vi "Keysight handler.vi"(8 "error in (no error)":errorcluster, 11 "Message Queues out":T1) -> (0 "error out":errorcluster, 3 "Message Queue":refnum<queue>)   [LabVIEW 2014]
uses:
  support/Message Queue/Message Queue.lvlib
  support/Message Queue/Enqueue Message (Single).vi
  <vilib>/ErrorRing/Error Ring.xnode
  support/Message Queue/Lossy Enqueue Message (Single).vi
  <vilib>/Utility/error.llb/Error Cluster From Error Code.vi
  Laser/Keyence data cluster.ctl
  Multimeter settings.ctl
  <instrlib>/Agilent 3446X Series/Public/Data/Read (Single Point).vi
  <vilib>/ethernetip/ethernetip.llb/ethernetip.ctl
  <vilib>/ethernetip/ethernetip.lvlib
  support/Message Queue/Message Cluster.ctl
  support/Message Queue/All Message Queues.ctl
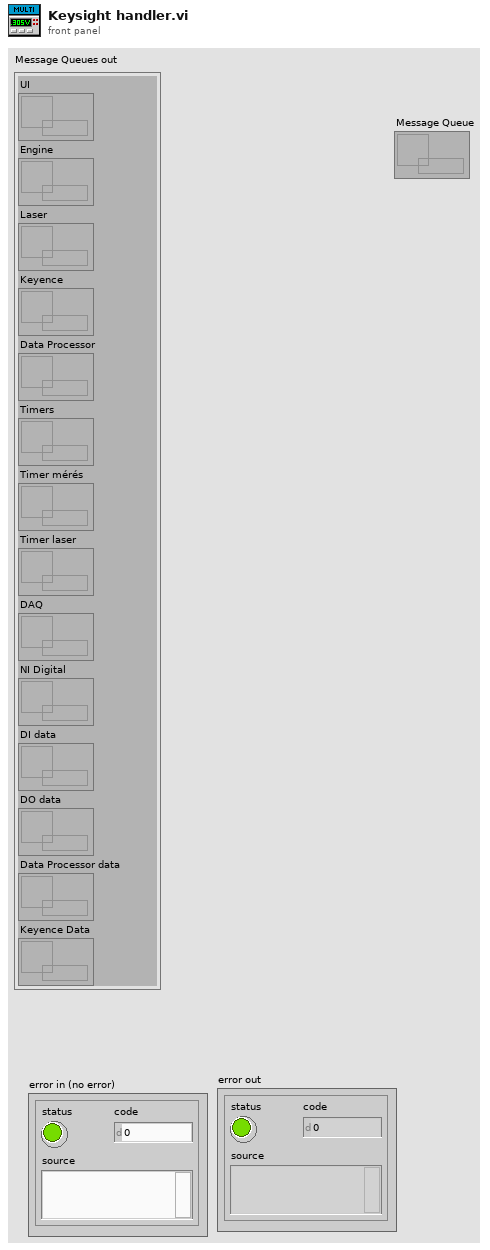
[diagram p1: front panel]
types:
  T1 = typedef "Message Queue.lvlib/All Message Queues.ctl" = cluster{"UI":refnum<queue>, "Engine":refnum<queue>, "Laser":refnum<queue>, "Keyence":refnum<queue>, "Data Processor":refnum<queue>, "Timers":refnum<queue>, "Timer mérés":refnum<queue>, "Timer laser":refnum<queue>, "DAQ":refnum<queue>, "NI Digital":refnum<queue>, "DI data":refnum<queue>, "DO data":refnum<queue>, "Data Processor data":refnum<queue>, "Keyence Data":refnum<queue>}
  T2 = typedef "Keyence data cluster.ctl" = cluster{"Communication Opened":bool, "Result":dbl[], "Read":bool, "Ethernet/IP Session":T3, "Ethernet/IP parameters":cluster{"IP":string, "Class":dbl, "Attribute":dbl, "Get Instance":dbl, "Set Instance":dbl}}
  T3 = typedef "ethernetip.lvlib/ethernetip.ctl" = refnum<k21>
  T4 = typedef "Multimeter settings.ctl" = cluster{"Measurement Function (10: Voltage DC)":i32, "Absolute Resolution (1E-6)":dbl, "Auto Range (T: Enable)":bool, "Manual Range (1)":dbl, "Command":string}
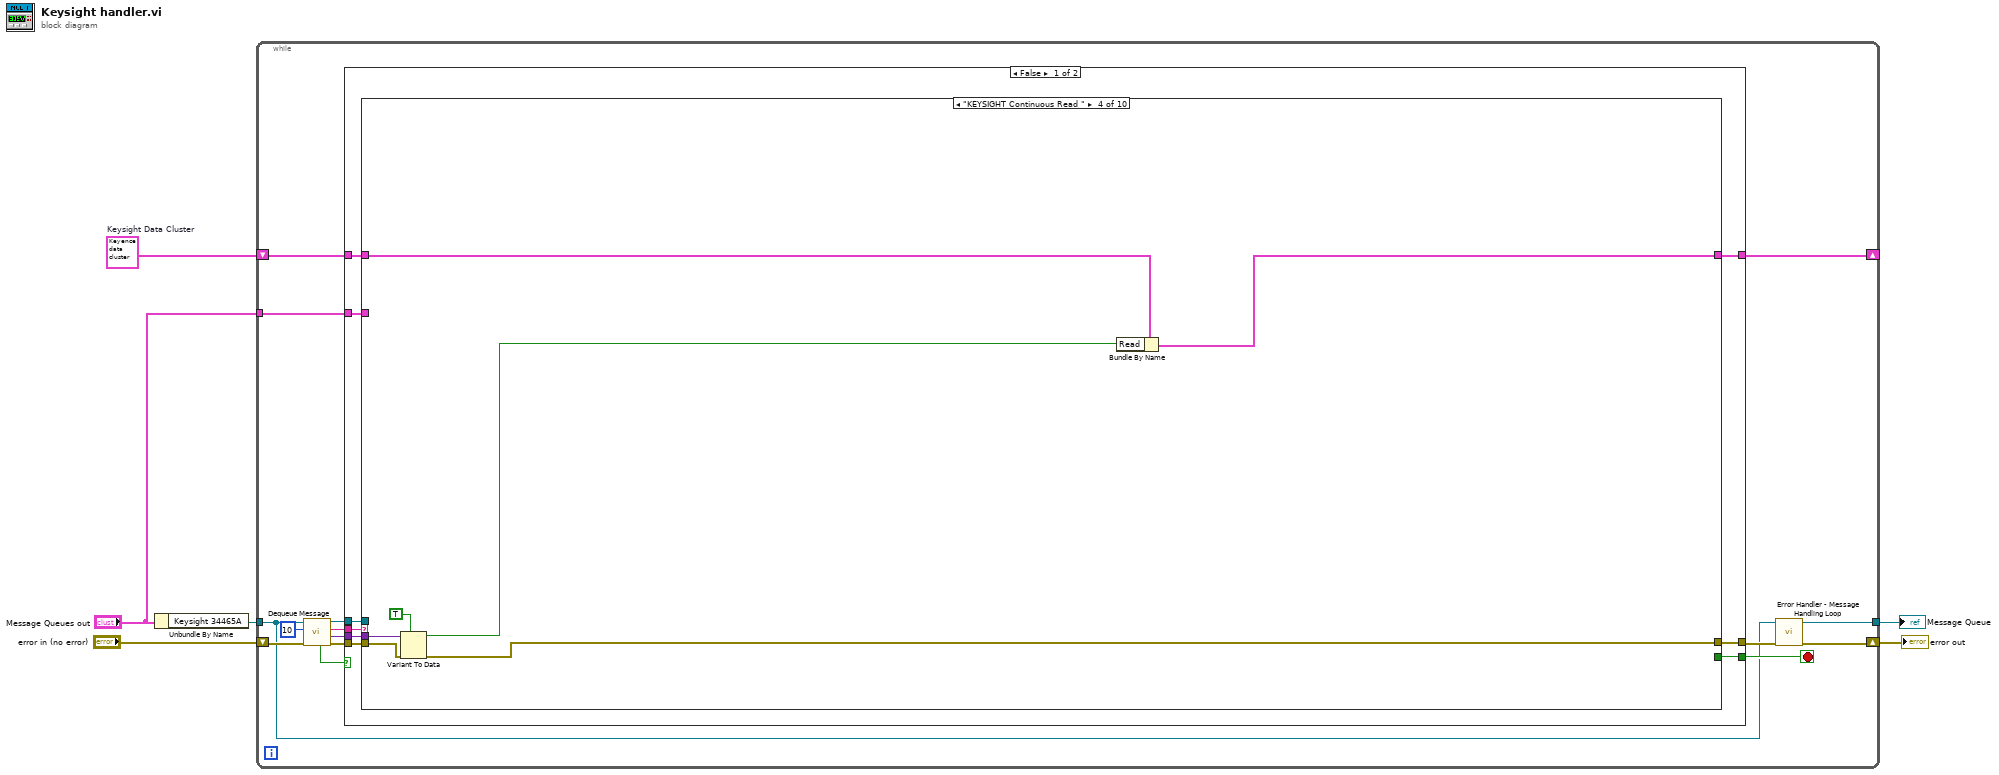
[diagram p0: block diagram]
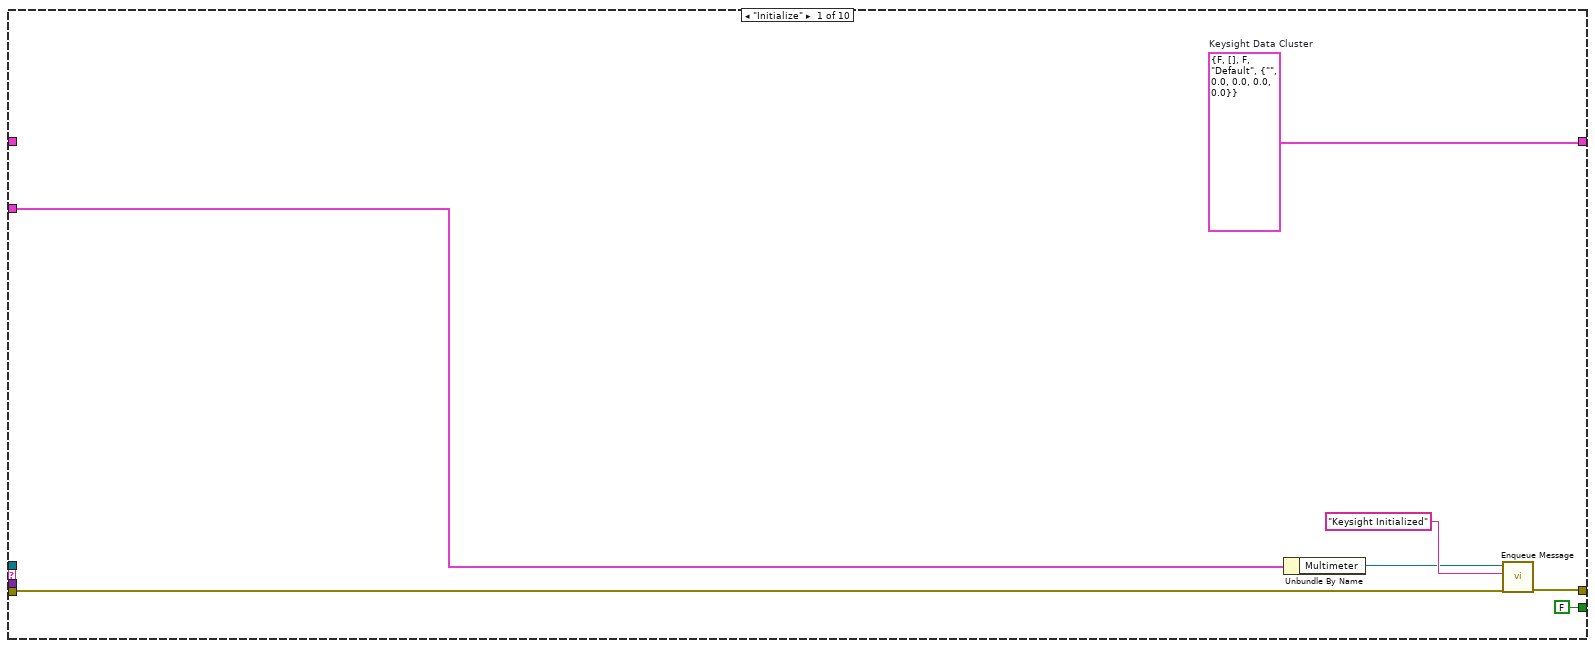
[diagram p2: hidden frame]
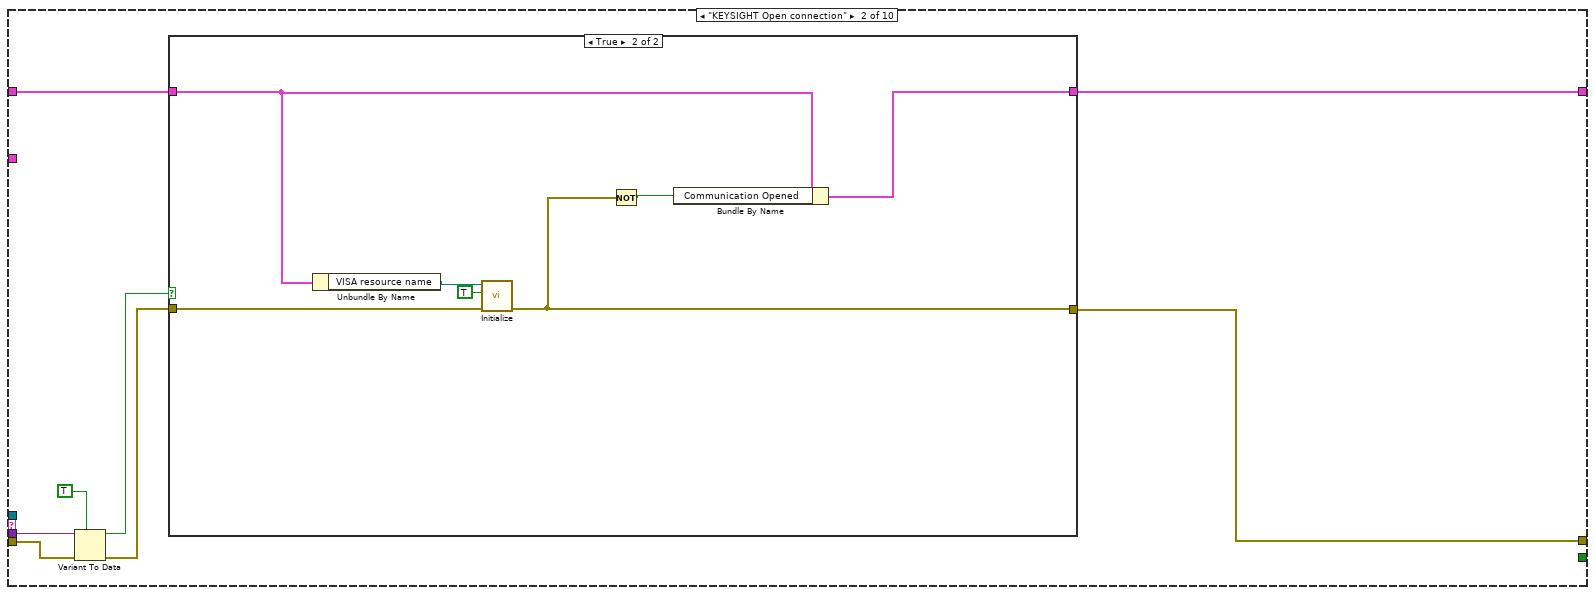
[diagram p3: hidden frame]
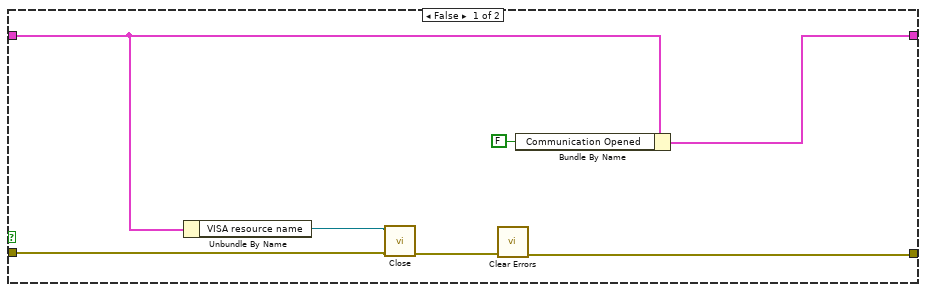
[diagram p4: hidden frame]
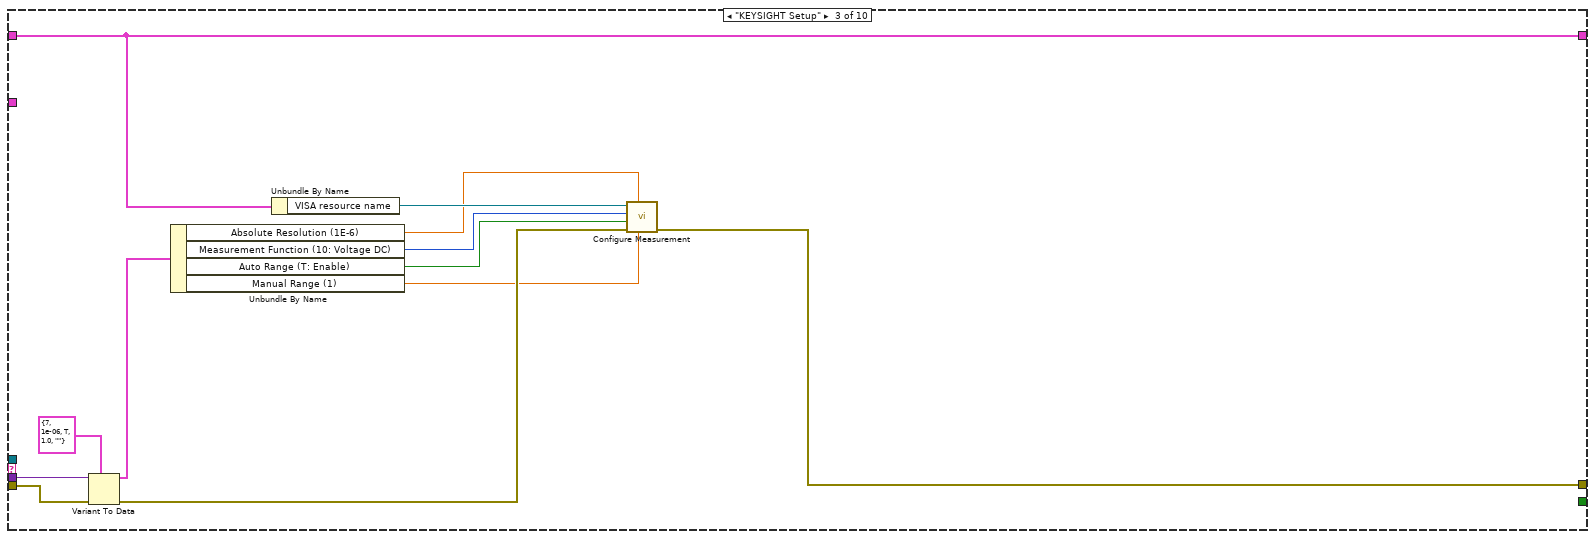
[diagram p5: hidden frame]
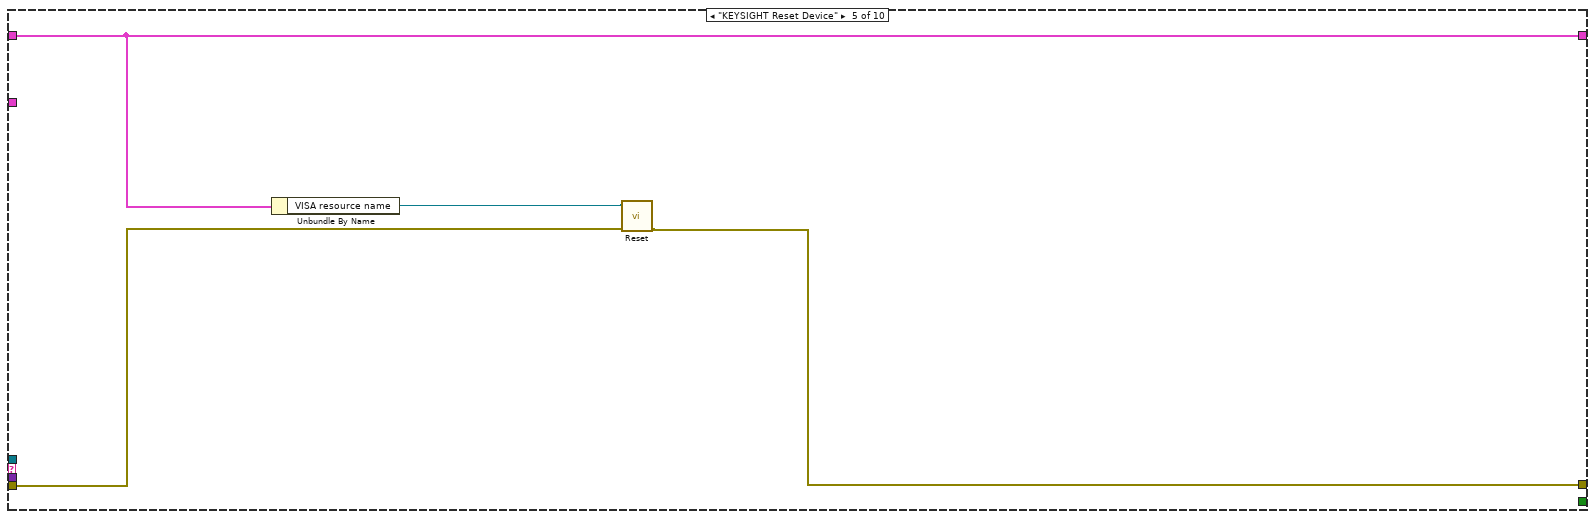
[diagram p6: hidden frame]
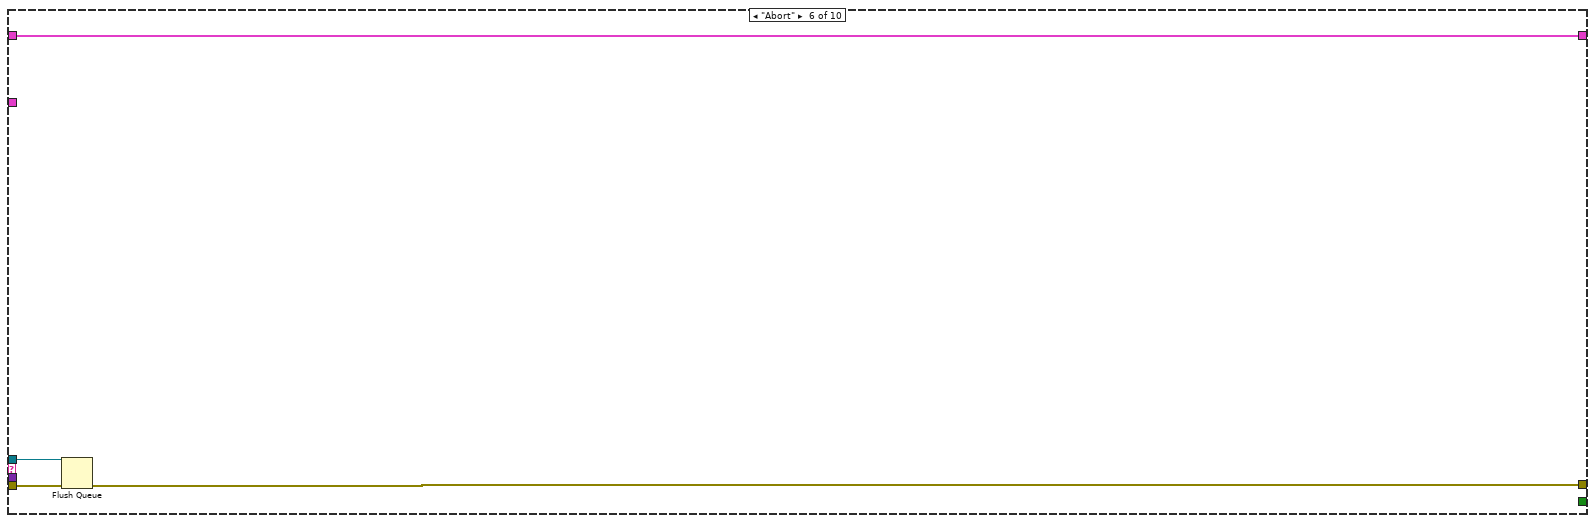
[diagram p7: hidden frame]
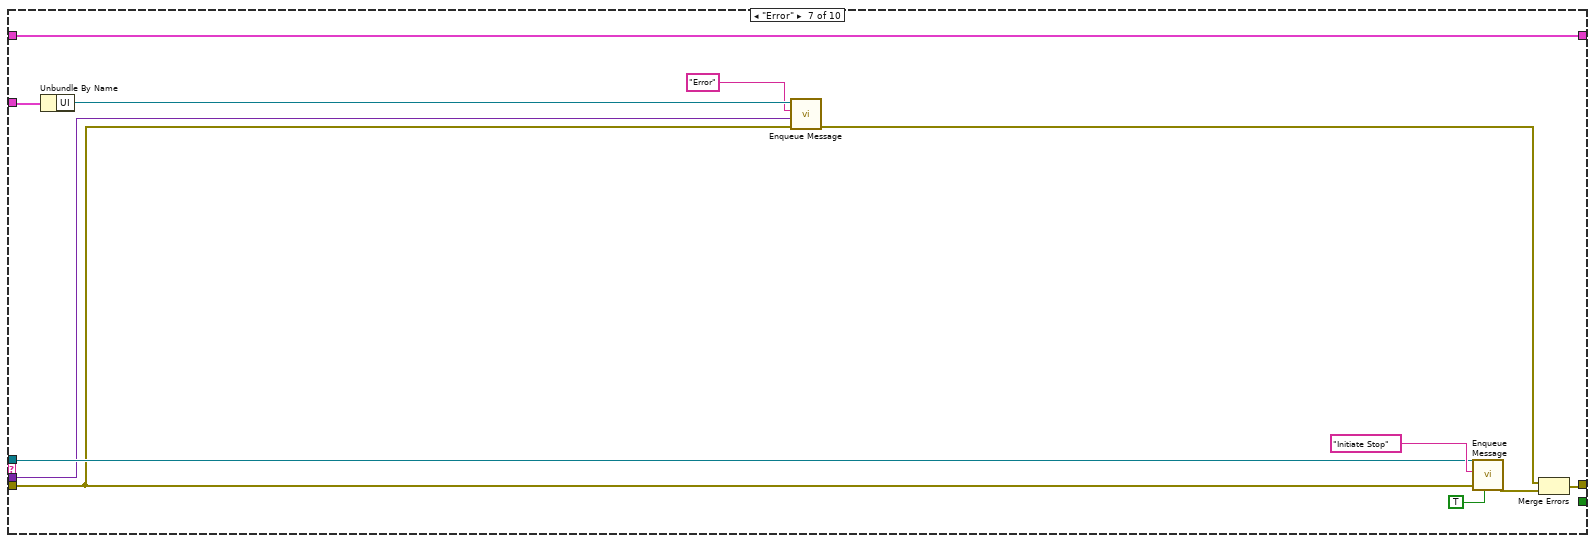
[diagram p8: hidden frame]
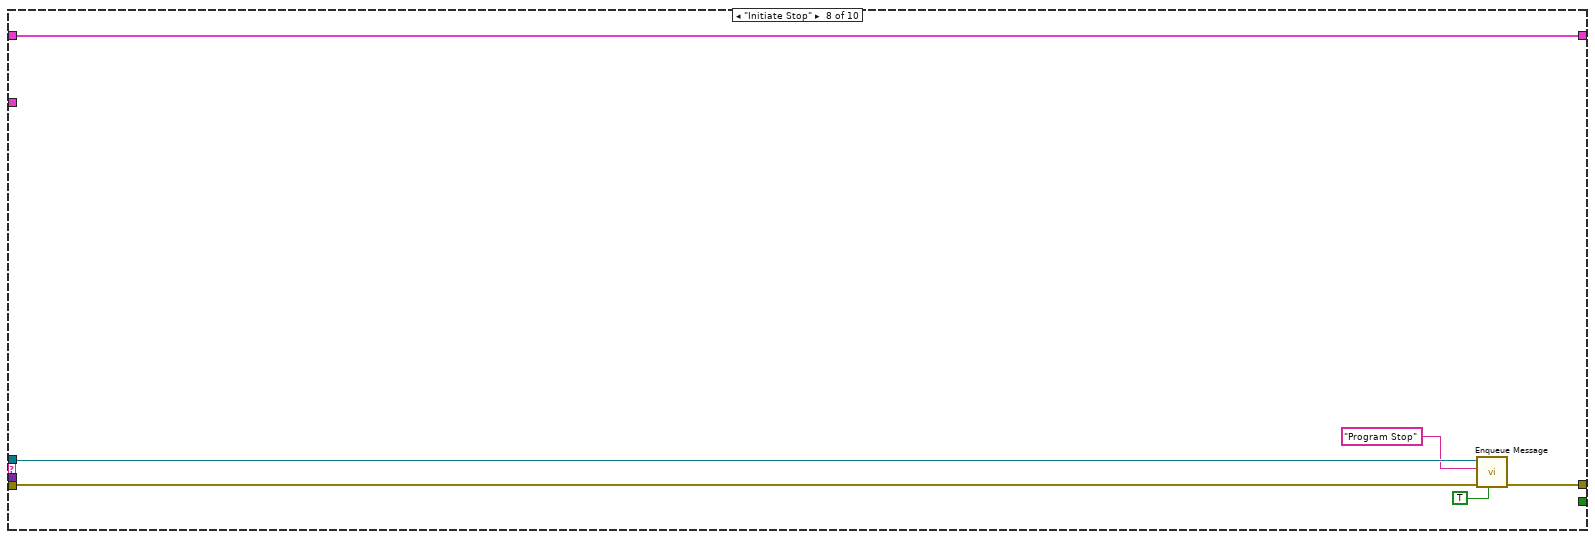
[diagram p9: hidden frame]
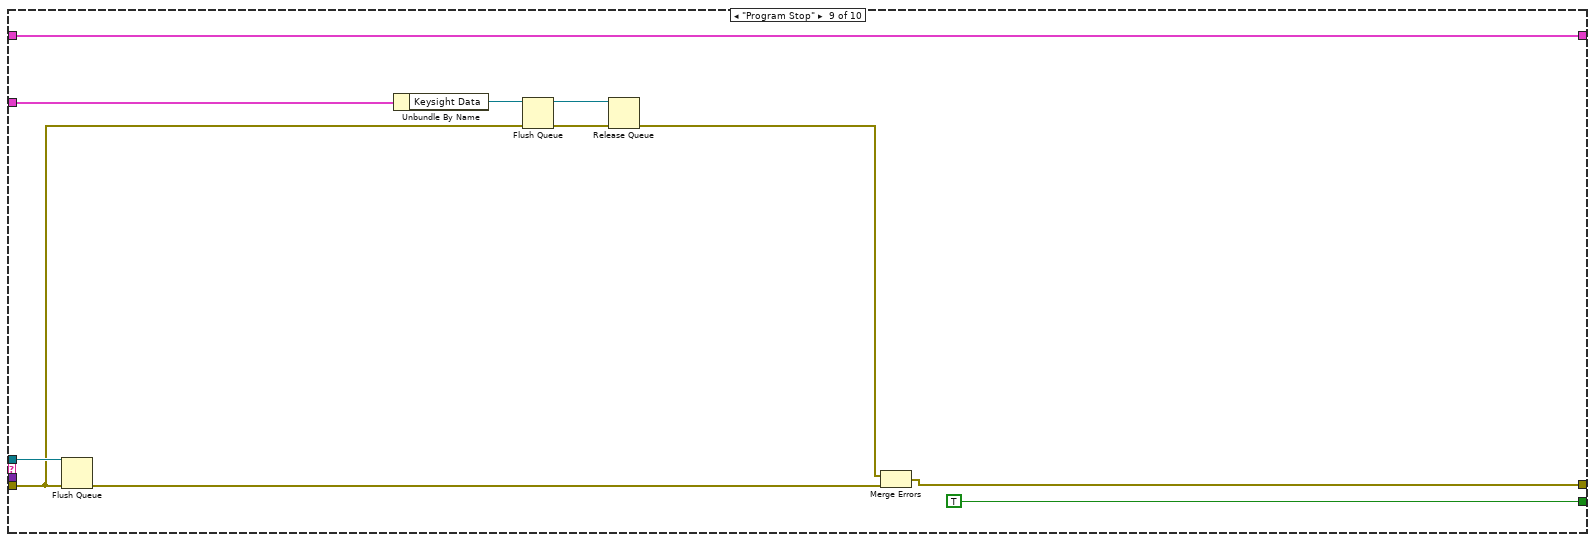
[diagram p10: hidden frame]
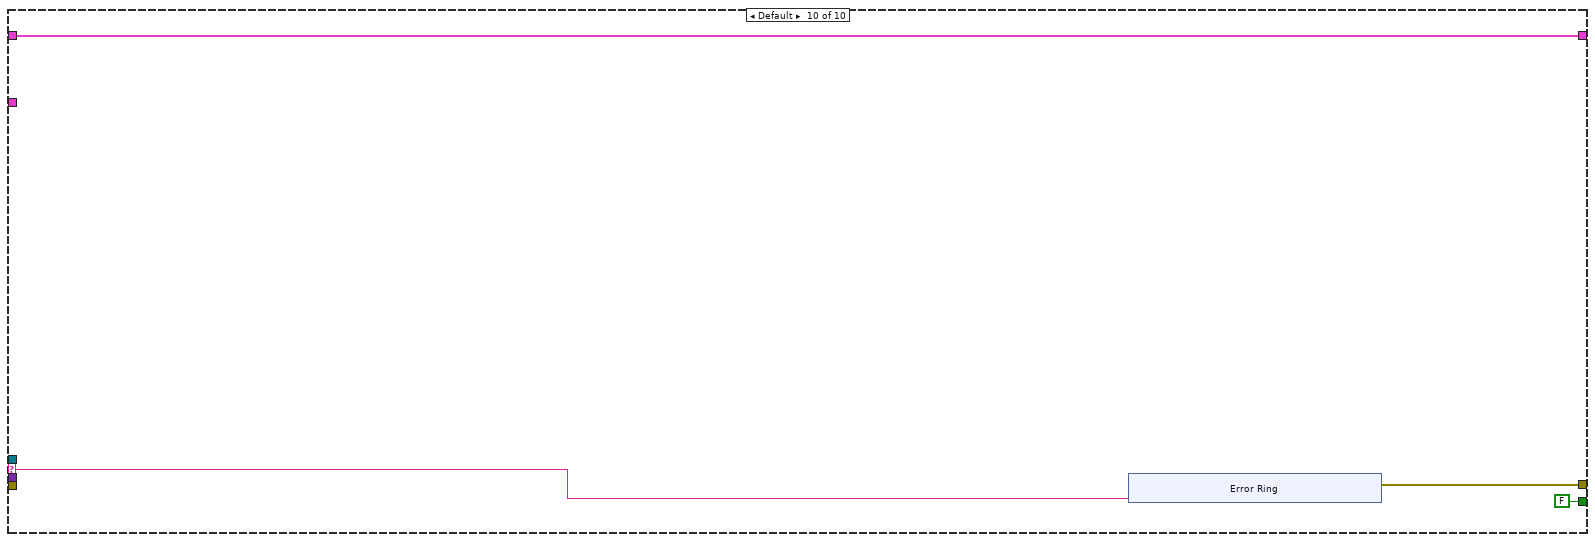
[diagram p11: hidden frame]
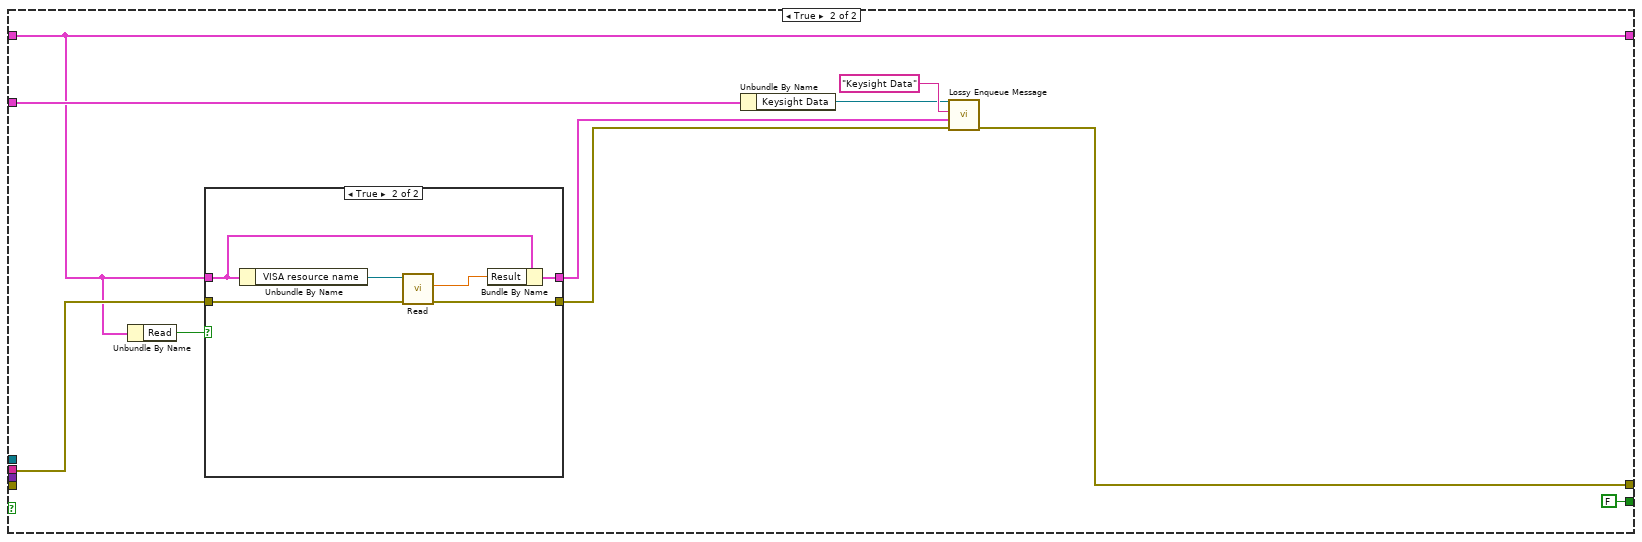
[diagram p12: hidden frame]
diagram:
  w1 = T2 {"Communication Opened"=FALSE, "Result"=[], "Read"=FALSE, "Ethernet/IP Session"="Default", "Ethernet/IP parameters"={"IP"="", "Class"=0.0, "Attribute"=0.0, "Get Instance"=0.0, "Set Instance"=0.0}}  # Keysight Data Cluster
  n1 = Unbundle By Name("Message Queues out") -> ("Keysight 34465A"=w3:refnum<queue>)
  n2 = while {
    tunnel: w3 -> [w7]
    shift-right: [w8] -> _
    shift-left: w1 -> [w14]
    shift-right: [w12] -> w6
    shift-left: "error in (no error)" -> [w21]
    tunnel: "Message Queues out" -> [w10]
    tunnel: [w9] -> w2
    stop <- w17 stop-if-true
    n3 = call "Dequeue Message.vi"("error in (no error)"=w21, "timeout in ms (-1)"=10, "Message Queue"=w7) -> ("error out"=w19:errorcluster, "Message Data"=w13:variant, "Message"=w20:string, "dup Message Queue"=w18:refnum<queue>, "timed out?"=w15:bool)  [unwired: 4 in]
    n4 = case shown="False" w15 {
      tunnel: w20 -> [w30 _]
      tunnel: w19 -> [w29 w131]
      tunnel: w18 -> [w28 _]
      tunnel: [w27 FALSE] -> w17
      tunnel: [w26 w132] -> w11
      tunnel: w14 -> [w24 w128]
      tunnel: [w25 w128] -> w8
      tunnel: w13 -> [w23 _]
      tunnel: w10 -> [w22 w133]
      frame False {
        n5 = case shown="\"KEYSIGHT Continuous Read \"" w30 {
          selector: w30 -> [_ _ _ _ _ _ _ _ _ w116]
          tunnel: w29 -> [w32 w41 w70 w75 w82 w86 w88 w102 w105 _]
          tunnel: w28 -> [_ _ _ _ _ w85 w91 w101 w115 _]
          tunnel: [w36 w38 w61 w72 w80 w83 w92 w103 w106 w117] -> w26
          tunnel: [FALSE _ _ _ _ _ _ _ TRUE FALSE] -> w27
          tunnel: [w31 w39 w60 w77 w79 w84 w87 w104 w113 w119] -> w25
          tunnel: w24 -> [_ w40 w60 w78 w79 w84 w87 w104 w113 w119]
          tunnel: w23 -> [_ w42 w71 w76 _ _ w89 _ _ _]
          tunnel: w22 -> [w33 _ _ _ _ _ w90 _ w108 _]
          frame "Initialize" {
            w31 = T2 {"Communication Opened"=FALSE, "Result"=[], "Read"=FALSE, "Ethernet/IP Session"="Default", "Ethernet/IP parameters"={"IP"="", "Class"=0.0, "Attribute"=0.0, "Get Instance"=0.0, "Set Instance"=0.0}}  # Keysight Data Cluster
            n6 = Unbundle By Name(w33) -> ("Multimeter"=w34:refnum<queue>)
            n7 = call-poly "Enqueue Message.vi"("error in (no error)"=w32, "Message"="Keysight Initialized", "Message Queue"=w34) -> ("error out"=w36:errorcluster)  [unwired: 7 in, 1 out]
          }
          frame "KEYSIGHT Open connection" {
            n8 = Variant To Data(error in=w41, type=TRUE ("Control word.Enable Voltage"), Variant=w42) -> (data=w43:bool, error out=w44:errorcluster)
            n9 = case shown="True" w43 {
              tunnel: w44 -> [w48 w59]
              tunnel: w40 -> [w52 w57]
              tunnel: [w50 w54] -> w38
              tunnel: [w49 w56] -> w39
              frame False {
                n10 = Unbundle By Name(w52) -> ("VISA resource name"=w46:refnum<visa-resource-name>)
                n11 = call <instrlib>:"Close.vi"("error in (no error)"=w48, "VISA resource name"=w46) -> ("error out"=w47:errorcluster)  [unwired: 9 in]
                n12 = call <vilib>:"Clear Errors.vi"("error in (no error)"=w47) -> ("error out"=w50:errorcluster)  [unwired: 5 in, 1 out]
                n13 = Bundle By Name(cluster=w52, "Communication Opened"=FALSE) -> (w49:T2)
              }
              frame True {
                n14 = Unbundle By Name(w57) -> ("VISA resource name"=w58:refnum<visa-resource-name>)
                n15 = call <instrlib>:"Initialize.vi"("error in (no error)"=w59, "ID Query (True)"=TRUE, "VISA resource name"=w58) -> ("error out"=w54:errorcluster)  [unwired: 7 in, 1 out]
                n16 = Not(x=w54) -> (.not. x?=w55:bool)
                n17 = Bundle By Name(cluster=w57, "Communication Opened"=w55) -> (w56:T2)
              }
            }
          }
          frame "KEYSIGHT Setup" {
            n18 = Variant To Data(error in=w70, type=T4 {"Measurement Function (10: Voltage DC)"=7, "Absolute Resolution (1E-6)"=1e-06, "Auto Range (T: Enable)"=TRUE, "Manual Range (1)"=1.0, "Command"=""} ("Multimeter settings"), Variant=w71) -> (data=w68:T4, error out=w66:errorcluster)
            n19 = Unbundle By Name(w68) -> ("Absolute Resolution (1E-6)"=w65:dbl, "Measurement Function (10: Voltage DC)"=w64:i32, "Auto Range (T: Enable)"=w63:bool, "Manual Range (1)"=w62:dbl)
            n20 = Unbundle By Name(w60) -> ("VISA resource name"=w67:refnum<visa-resource-name>)
            n21 = call <instrlib>:"Configure Measurement.vi"("Manual Range (1)"=w62, "Absolute Resolution (1E-6)"=w65, "error in (no error)"=w66, "Auto Range (T: Enable)"=w63, "Measurement Function (10: Voltage DC)"=w64, "VISA resource name"=w67) -> ("error out"=w61:errorcluster)  [unwired: 4 in, 1 out]
          }
          frame "KEYSIGHT Continuous Read " {
            n22 = Variant To Data(error in=w75, type=TRUE, Variant=w76) -> (data=w73:bool, error out=w72:errorcluster)
            n23 = Bundle By Name(cluster=w78, "Read"=w73) -> (w77:T2)
          }
          frame "KEYSIGHT Reset Device" {
            n24 = Unbundle By Name(w79) -> ("VISA resource name"=w81:refnum<visa-resource-name>)
            n25 = call <instrlib>:"Reset.vi"("error in (no error)"=w82, "VISA resource name"=w81) -> ("error out"=w80:errorcluster)  [unwired: 8 in, 1 out]
          }
          frame "Abort" {
            n26 = Flush Queue(queue=w85, error in (no error)=w86) -> (error out=w83:errorcluster)  [unwired: 2 out]
          }
          frame "Error" {
            n27 = Unbundle By Name(w90) -> ("UI"=w95:refnum<queue>)
            n28 = call-poly "Enqueue Message.vi"("error in (no error)"=w88, "Message Data"=w89, "Message"="Error", "Message Queue"=w95) -> ("error out"=w97:errorcluster)  [unwired: 6 in, 1 out]
            n29 = call-poly "Enqueue Message.vi"("Priority Message? (F)"=TRUE, "error in (no error)"=w88, "Message"="Initiate Stop", "Message Queue"=w91) -> ("error out"=w96:errorcluster)  [unwired: 6 in, 1 out]
            n30 = Merge Errors(w97, w96) -> (w92:errorcluster)
          }
          frame "Initiate Stop" {
            n31 = call-poly "Enqueue Message.vi"("Priority Message? (F)"=TRUE, "error in (no error)"=w102, "Message"="Program Stop", "Message Queue"=w101) -> ("error out"=w103:errorcluster)  [unwired: 6 in, 1 out]
          }
          frame "Program Stop" {
            n32 = Flush Queue(queue=w115, error in (no error)=w105) -> (error out=w107:errorcluster)  [unwired: 2 out]
            n33 = Unbundle By Name(w108) -> ("Keysight Data"=w109:refnum<queue>)
            n34 = Flush Queue(queue=w109, error in (no error)=w105) -> (queue out=w110:refnum<queue>, error out=w111:errorcluster)  [unwired: 1 out]
            n35 = Release Queue(queue=w110, error in (no error)=w111) -> (error out=w112:errorcluster)  [unwired: 1 in, 2 out]
            n36 = Merge Errors(w112, w107) -> (w106:errorcluster)
          }
          frame Default {
            n37 = xnode "Error Ring"("parameter 0"=w116) -> ("error out"=w117:errorcluster)
          }
        }
      }
      frame True {
        n38 = Unbundle By Name(w128) -> ("Read"=w127:bool)
        n39 = case shown="True" w127 {
          tunnel: w131 -> [w137 w144]
          tunnel: w128 -> [w138 w142]
          tunnel: [w137 w140] -> w130
          tunnel: [w138 w139] -> w129
          frame False {
          }
          frame True {
            n40 = Unbundle By Name(w142) -> ("VISA resource name"=w143:refnum<visa-resource-name>)
            n41 = call-poly <instrlib>:"Read.vi"("error in (no error)"=w144, "VISA resource name"=w143) -> ("error out"=w140:errorcluster, "Measurement"=w141:dbl)  [unwired: 7 in, 1 out]
            n42 = Bundle By Name(cluster=w142, "Result"=w141) -> (w139:T2)
          }
        }
        n43 = Unbundle By Name(w133) -> ("Keysight Data"=w134:refnum<queue>)
        n44 = call-poly "Lossy Enqueue Message.vi"("error in (no error)"=w130, "Message Data"=w129, "Message"="Keysight Data", "Message Queue"=w134) -> ("error out"=w132:errorcluster)  [unwired: 6 in, 1 out]
      }
    }
    n45 = call "Error Handler - Message Handling Loop.vi"("error in (no error)"=w11, "Message Queue"=w7) -> ("dup error in"=w12:errorcluster, "dup Message Queue"=w9:refnum<queue>)  [unwired: 8 in]
  }
  "error out" <- w6
  "Message Queue" <- w2
